vi "Format By List Image Description Rows.vi"(4 "Width (500 pixels)":i16=500, 6 "Image":path, 8 "error in (no error)":errorcluster {"code" format="Error %.0f"}, 9 "Description":string, 10 "Name":string, 11 "VIDoc Printer - Confluence In":refnum<class "VIDoc Printer - Confluence.lvclass">) -> (0 "error out":errorcluster {"code" format="Error %.0f"}, 1 "Table Headers":string[](array[string]), 2 "Table Rows Text":string, 3 "VIDoc Printer - Confluence Out":refnum<class "VIDoc Printer - Confluence.lvclass">)   [LabVIEW 2023, in "VIDoc Printer - Confluence.lvlib" / "VIDoc Printer - Confluence.lvclass"]
uses:
  VIDoc Printer - Confluence.lvclass
  VIDoc Printer - Confluence.lvclass/VIDoc Printer - Confluence.ctl
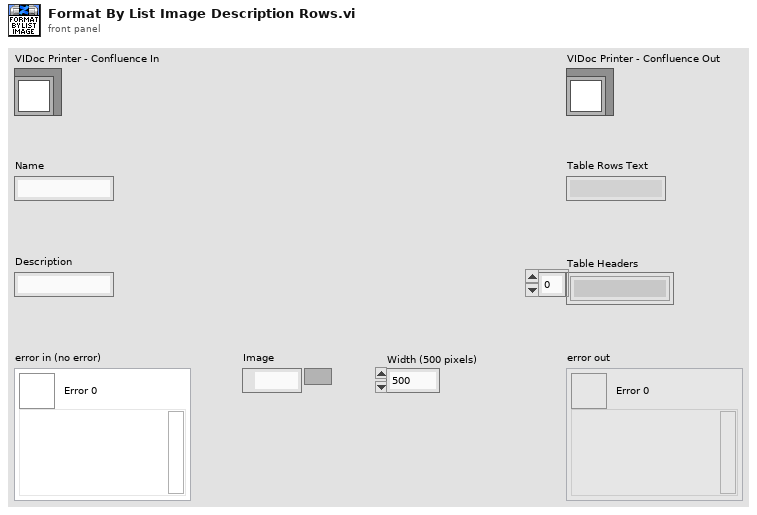
[diagram p1: front panel]
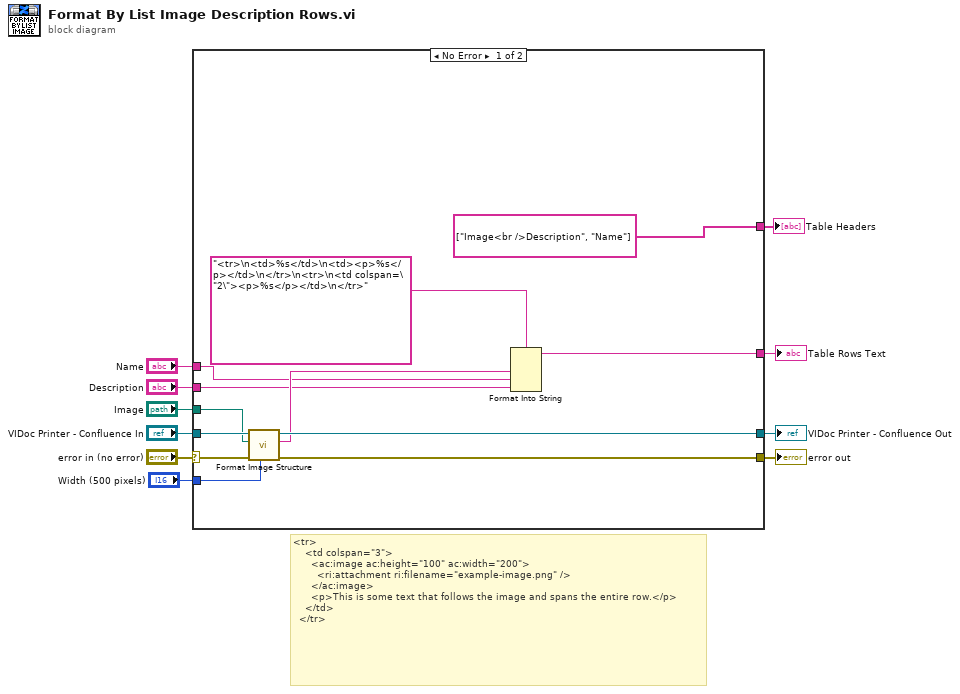
[diagram p0: block diagram]
diagram:
  # "<tr>\n    <td colspan=\"3\">\n      <ac:image ac:height=\"100\" ac:width=\"200\">\n        <ri:attachment ri:filename=\"example-image.png\" />\n      </ac:image>\n      <p>This is some text that follows the image and spans the entire row.</p>\n    </td>\n  </tr>"
  n1 = case shown="No Error" "error in (no error)" {
    selector: "error in (no error)" -> [w20 w24]
    tunnel: [w19 w24] -> w9
    tunnel: [w22 w23] -> w7
    tunnel: "VIDoc Printer - Confluence In" -> [w21 w23]
    tunnel: "Image" -> [w18 _]
    tunnel: "Description" -> [w16 _]
    tunnel: [w15 _] -> w4
    tunnel: "Name" -> [w14 _]
    tunnel: "Width (500 pixels)" -> [w13 _]
    tunnel: [string[] ["Image<br />Description", "Name"] ("Table Headers") _] -> w1
    frame No Error {
      n2 = call "Format Image Structure.vi"("Max Width (500 pixels)"=w13, "error in (no error)"=w20, "Image"=w18, "VIDoc Printer - Confluence In"=w21) -> ("error out"=w19:errorcluster, "Image Structure Text"=w17:string, "VIDoc Printer - Confluence Out"=w22:refnum<class "VIDoc Printer - Confluence.lvclass">)  [unwired: 5 in]
      n3 = Format Into String(format string="<tr>\n<td>%s</td>\n<td><p>%s</p></td>\n</tr>\n<tr>\n<td colspan=\"2\"><p>%s</p></td>\n</tr>", w17, w14, w16) -> (resulting string=w15:string)  [unwired: 2 in, 1 out]
    }
    frame Error {
    }
  }
  "error out" <- w9
  "VIDoc Printer - Confluence Out" <- w7
  "Table Rows Text" <- w4
  "Table Headers" <- w1
